vi "Terminal-PressureSystemDeviceLubricateUnit-Setter.vi"(8 "error in (no error)":errorcluster caption="错误输入（无错误）", 10 "启停":bool=TRUE, 11 "operation timeout (ms)":i32=5000 caption="操作超时（5000毫秒）") -> (0 "error out":errorcluster caption="错误输出")   [LabVIEW 2014]
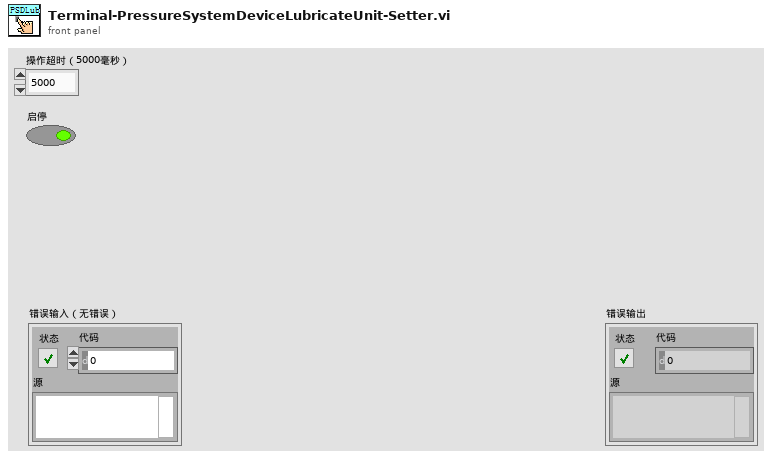
[diagram p1: front panel]
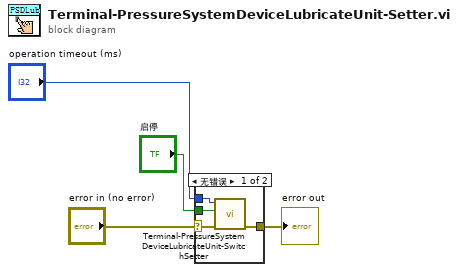
[diagram p0: block diagram]
diagram:
  n1 = case shown="无错误" "error in (no error)" {
    selector: "error in (no error)" -> [w7 w9]
    tunnel: "operation timeout (ms)" -> [w5 _]
    tunnel: [w8 w9] -> w3
    tunnel: "启停" -> [w6 _]
    frame No Error {
      n2 = call "Terminal-PressureSystemDeviceLubricateUnit-SwitchSetter.vi"("error in (no error)"=w7, "启停"=w6, "operation timeout (ms)"=w5) -> ("error out"=w8:errorcluster)  [unwired: 8 in]
    }
    frame Error {
    }
  }
  "error out" <- w3
